vi "_Possible State Owner.vi"(11 "regular expression":string=">>") -> (1 "owners":string[](array[string]), 3 "state":string)   [LabVIEW 2017]
uses:
  <vilib>/Utility/config.llb/Close Config Data.vi
  <vilib>/Utility/config.llb/Get Section Names.vi
  <vilib>/Utility/config.llb/Open Config Data.vi
  _csmHelper/lvcsmFile/lvcsm File Path.vi
  _csmHelper/lvcsmFile/lvcsm File Support.lvlib
  <vilib>/regexp/Match Regular Expression.xnode
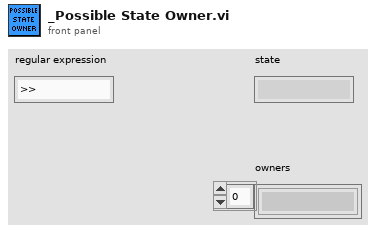
[diagram p1: front panel]
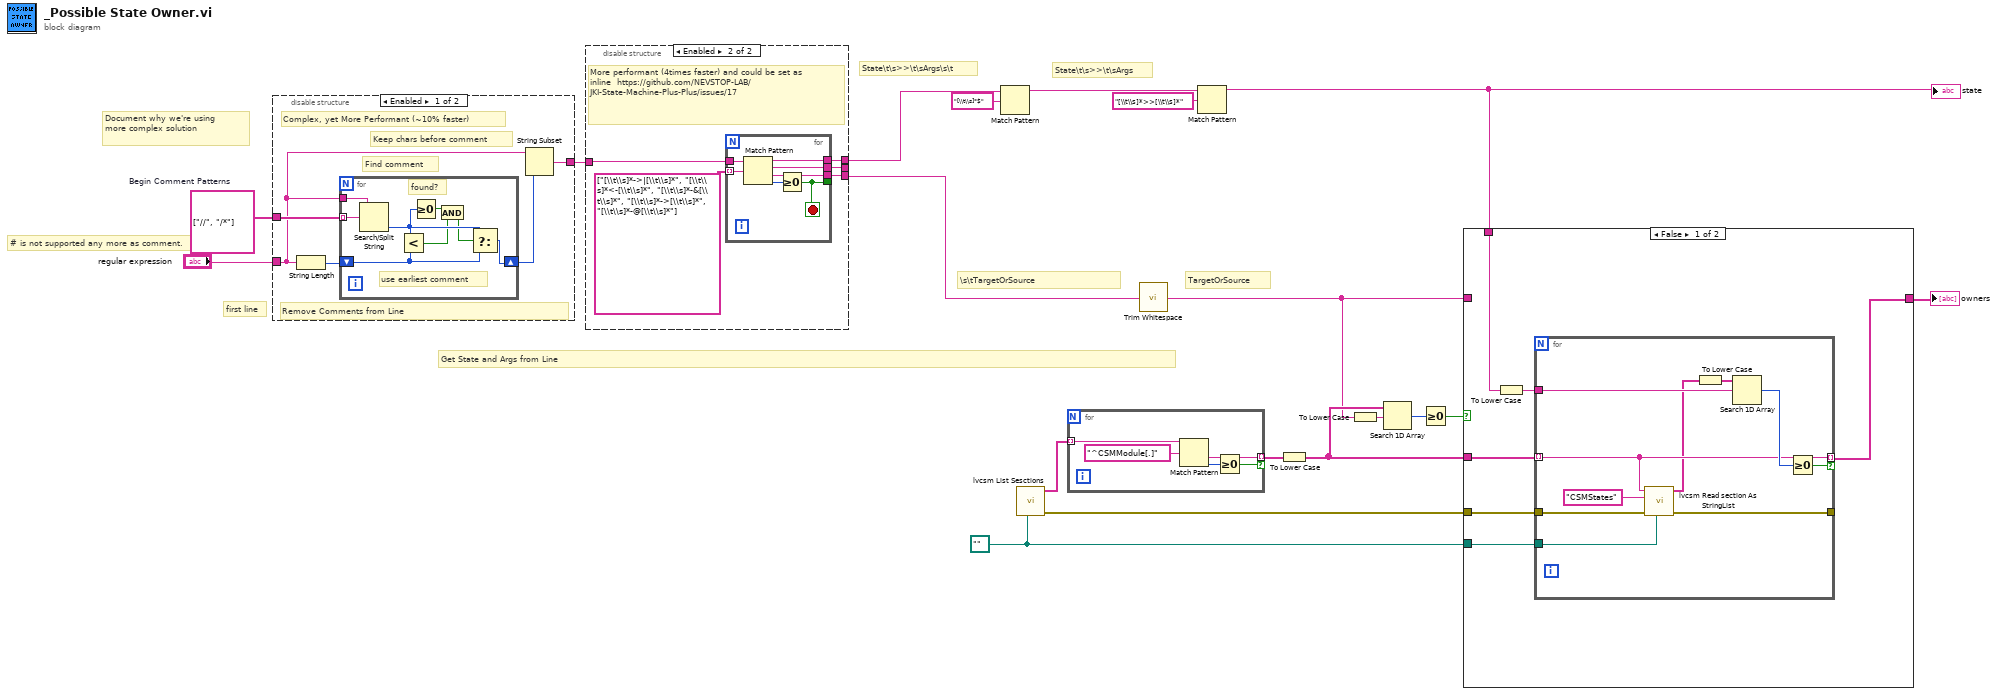
[diagram p0: block diagram]
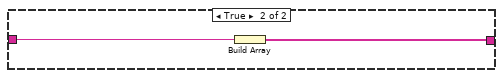
[diagram p2: hidden frame]
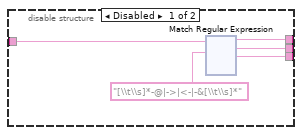
[diagram p3: hidden frame]
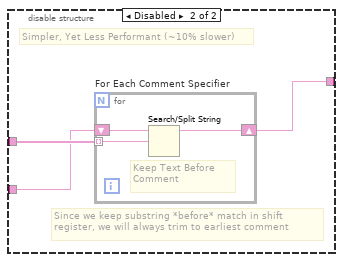
[diagram p4: hidden frame]
diagram:
  w9 = path "" ("Config Path(\"\" for lvcsm file)")
  w19 = string[] ["//", "/*"]  # Begin Comment Patterns
  # "TargetOrSource"
  # "State\\t\\s>>\\t\\sArgs"
  # "State\\t\\s>>\\t\\sArgs\\s\\t"
  # "Get State and Args from Line"
  # "\\s\\tTargetOrSource"
  # "# is not supported any more as comment."
  # "Document why we're using more complex solution"
  # "first line"
  n1 = disable-structure "Diagram Disable Structure" shown="Enabled" {
    disable-tunnel: w19 -> [w24 w35]
    disable-tunnel: [w23 w34] -> w13
    disable-tunnel: "regular expression" -> [w22 w33]
    frame Enabled {
      # "Remove Comments from Line"
      # "Complex, yet More Performant (~10% faster)"
      # "Keep chars before comment"
      # "Find comment"
      n2 = String Length(string=w22) -> (length=w21:i32)
      n3 = for {
        tunnel: w24 -> [w29] mode=indexing
        shift-right: [w31] -> w20
        shift-left: w21 -> [w32]
        tunnel: w22 -> [w30]
        # "found?"
        # "use earliest comment"
        n4 = Search/Split String(string=w30, search string/char (-)=w29) -> (offset of match=w28:i32)  [unwired: 1 in, 2 out]
        n5 = Less?(x=w28, y=w32) -> (x < y?=w26:bool)
        n6 = Greater Or Equal To 0?(x=w28) -> (x >= 0?=w27:bool)
        n7 = And(x=w27, y=w26) -> (x .and. y?=w25:bool)
        n8 = Select(t=w28, s=w25, f=w32) -> (s? t:f=w31:i32)
      }
      n9 = String Subset(string=w22, length (rest)=w20) -> (substring=w23:string)  [unwired: 1 in]
    }
    frame Disabled {
      # "Since we keep substring *before* match in shift register, we will always trim to earliest comment"
      # "Simpler, Yet Less Performant (~10% slower)"
      n10 = for "For Each Comment Specifier" {
        tunnel: w35 -> [w37] mode=indexing
        shift-right: [w36] -> w34
        shift-left: w33 -> [w38]
        # "Keep Text Before Comment"
        n11 = Search/Split String(string=w38, search string/char (-)=w37) -> (substring before match=w36:string)  [unwired: 1 in, 2 out]
      }
    }
  }
  n12 = disable-structure shown="Enabled" {
    disable-tunnel: [w42 w160] -> w15
    disable-tunnel: [w41 w159] -> _
    disable-tunnel: [w40 w158] -> w2
    disable-tunnel: w13 -> [w39 w162]
    frame Disabled {
      n13 = xnode "Match Regular Expression"("input string"=w39, "regular expression"="[\\t\\s]*-@|->|<-|-&[\\t\\s]*") -> ("before match"=w42:string, "whole match"=w41:string, "after match"=w40:string)  [unwired: 4 in, 2 out]
    }
    frame Enabled {
      # "More performant (4times faster) and could be set as inline  https://github.com/NEVSTOP-LAB/JKI-State-Machine-Plus-Plus/issues/17"
      n14 = for {
        tunnel: w162 -> [w169]
        tunnel: string[] ["[\\t\\s]*->|[\\t\\s]*", "[\\t\\s]*<-[\\t\\s]*", "[\\t\\s]*-&[\\t\\s]*", "[\\t\\s]*->[\\t\\s]*", "[\\t\\s]*-@[\\t\\s]*"] -> [w168] mode=indexing
        tunnel: [w166] -> _
        tunnel: [w165] -> w160
        tunnel: [w164] -> w159
        tunnel: [w163] -> w158
        stop <- w166 stop-if-true
        n15 = Match Pattern(string=w169, regular expression=w168) -> (before substring=w165:string, match substring=w164:string, after substring=w163:string, offset past match=w167:i32)  [unwired: 1 in]
        n16 = Greater Or Equal To 0?(x=w167) -> (x >= 0?=w166:bool)
      }
    }
  }
  n17 = Match Pattern(string=w15, regular expression="[\\t\\s]*$") -> (before substring=w14:string)  [unwired: 1 in, 3 out]
  n18 = call "lvcsm List Sesctions.vi"("Config Path"=w9) -> ("Error out"=w10:errorcluster, "section names"=w11:string[])  [unwired: 9 in]
  n19 = for {
    tunnel: w11 -> [w174] mode=indexing
    tunnel: [w172] -> w8 mode=indexing if=w171
    n20 = Match Pattern(string=w174, regular expression="^CSMModule[.]" ("Section")) -> (after substring=w172:string, offset past match=w170:i32)  [unwired: 1 in, 2 out]
    n21 = Greater Or Equal To 0?(x=w170) -> (x >= 0?=w171:bool)
  }
  n22 = call <vilib>:"Trim Whitespace.vi"("string"=w2) -> ("trimmed string"=w1:string)  [unwired: 1 in]
  n23 = Match Pattern(string=w14, regular expression="[\\t\\s]*>>[\\t\\s]*") -> (before substring=w12:string)  [unwired: 1 in, 3 out]
  "state" <- w12
  n24 = To Lower Case(string=w8) -> (all lower case string=w7:string[])
  n25 = To Lower Case(string=w1) -> (all lower case string=w6:string)
  n26 = Search 1D Array(1D array=w7, element=w6) -> (index of element=w5:i32)  [unwired: 1 in]
  n27 = Greater Or Equal To 0?(x=w5) -> (x >= 0?=w4:bool)
  n28 = case shown="False" w4 {
    tunnel: w12 -> [w180 _]
    tunnel: w10 -> [w179 _]
    tunnel: w9 -> [w177 _]
    tunnel: w7 -> [w176 _]
    tunnel: [w175 w191] -> w3
    tunnel: w1 -> [_ w192]
    frame False {
      n29 = To Lower Case(string=w180) -> (all lower case string=w178:string)
      n30 = for {
        tunnel: w176 -> [w184] mode=indexing
        tunnel: [w184] -> w175 mode=indexing if=w188
        tunnel: w178 -> [w185]
        tunnel: w177 -> [w186]
        tunnel: w179 -> [w190]
        tunnel: [w189] -> _
        n31 = call "lvcsm Read section As StringList.vi"("Config Path(\"\" for lvcsm file)"=w186, "error in (no error)"=w190, "API Name"="CSMStates", "CSM Name"=w184) -> ("Error out"=w189:errorcluster, "CSMAPI List"=w182:string[])  [unwired: 6 in]
        n32 = To Lower Case(string=w182) -> (all lower case string=w181:string[])
        n33 = Search 1D Array(1D array=w181, element=w185) -> (index of element=w187:i32)  [unwired: 1 in]
        n34 = Greater Or Equal To 0?(x=w187) -> (x >= 0?=w188:bool)
      }
    }
    frame True {
      n35 = Build Array(w192) -> (w191:string[])
    }
  }
  "owners" <- w3
